vi "Memory.Pointer.U8.New.vi"(8 "error in (no error)":errorcluster) -> (0 "error out":errorcluster, 3 "U8 Pointer":refnum<class "Memory.Pointer.U8.lvclass">)   [LabVIEW 2016, in "Memory Manager.lvlib" / "Memory.Pointer.U8.lvclass"]
doc: "Allocates a new block of memory, represented by Pointer."
uses:
  Memory.Pointer.U8.lvclass
  Pointer.Numeric/Memory.Pointer.Numeric.lvclass/Memory.Pointer.Numeric.ctl
  Pointer.Void/Memory.Pointer.Void.lvclass/Memory.Pointer.Void.ctl
  Pointer.Numeric/Methods/Memory.Pointer.Numeric.Set power of 2.vi
  Pointer.Void/Methods/Memory.Pointer.Allocate.vi
  Pointer.Void/Methods/Memory.Pointer.Set Size.vi
  Pointer.Void/Methods/Memory.Pointer.Set Address.vi
  Pointer.Void/Methods/Memory.Pointer.Get Size.vi
  Pointer.Numeric/Memory.Pointer.Numeric.lvclass
  C:/Users/Ryan/Documents/Git/Sourcetree/LabVIEW-Memory-Manager/Source/Library/Classes/Pointer/Pointer.Void/Memory.Pointer.Void.lvclass
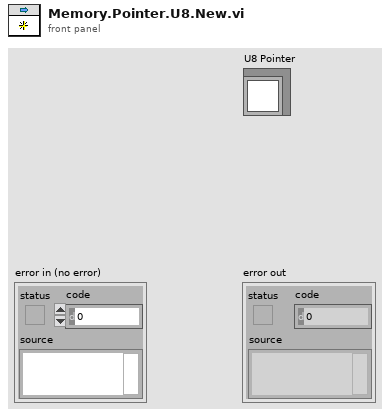
[diagram p1: front panel]
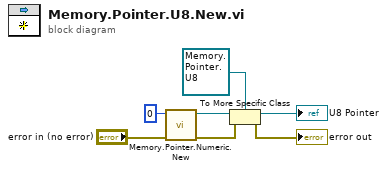
[diagram p0: block diagram]
diagram:
  n1 = call "Memory.Pointer.Numeric.New.vi"("error in (no error)"="error in (no error)", "power of 2"=i16 0) -> ("error out"=w5:errorcluster, "Numeric Pointer out"=w6:refnum<class "Memory.Pointer.Numeric.lvclass">)  [unwired: 8 in]
  n2 = To More Specific Class(target class=refnum<class "Memory.Pointer.U8.lvclass"> refnum ("LabVIEW Memory Manager.lvlib:DBL Pointer"), reference=w6, error in=w5) -> (specific class reference=→"U8 Pointer":refnum<class "Memory.Pointer.U8.lvclass">, error out=→"error out":errorcluster)
